vi "Int16 Encode.vi"(11 "数值":u16) -> (3 "数组":u8[](array[numeric]))   [LabVIEW 2016, in "DGUS.lvlib" / "DGUS.lvclass"]
uses:
  DGUS.lvclass
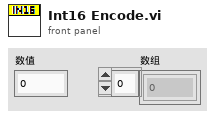
[diagram p1: front panel]
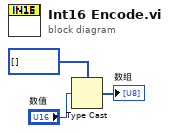
[diagram p0: block diagram]
diagram:
  n1 = Type Cast(type=u8[] [] ("数组"), x="数值") -> (*(type *) &x=→"数组":u8[])
